vi "Enum Shunt to Gain.vi"(1 "Shunt Resistor":T1) -> (0 "Gain (V/A)":dbl)   [LabVIEW 2019, in "KH7008.lvlib"]
uses:
  KH7008.lvlib
  typedefs/shunt--enum.ctl
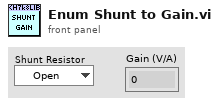
[diagram p1: front panel]
types:
  T1 = typedef "KH7008.lvlib/shunt--enum.ctl" = enum16{"Open", "50", "500", "5k", "50k", "10M"}
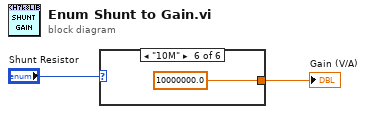
[diagram p0: block diagram]
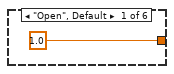
[diagram p2: hidden frame]
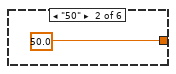
[diagram p3: hidden frame]
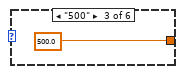
[diagram p4: hidden frame]
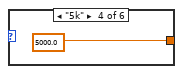
[diagram p5: hidden frame]
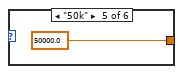
[diagram p6: hidden frame]
diagram:
  n1 = case shown="\"10M\"" "Shunt Resistor" {
    tunnel: [1.0 ("y") 50.0 ("y") 500.0 ("y") 5000.0 ("y") 50000.0 ("y") 10000000.0 ("y")] -> w1
    frame "Open", Default {
    }
    frame "50" {
    }
    frame "500" {
    }
    frame "5k" {
    }
    frame "50k" {
    }
    frame "10M" {
    }
  }
  "Gain (V/A)" <- w1
